vi "XML Script - GrowableNode (Style String).vi"(0 "x":i32=-1, 1 "y":i32=-1, 2 "out":i32=-1, 4 "Growable Node Style":string, 6 "name":string, 8 "size":i32=1, 9 "prefix (name)":string, 10 "in":i32=-1) -> (5 "name (wire source)":string, 7 "XML Script Command - Growable Node":string)   [LabVIEW 2017]
uses:
  <vilib>/_script/XML Scripting/XML Script Attribute.ctl
  <vilib>/_script/XML Scripting/XML Script Tag.ctl
panel:
  # "position"
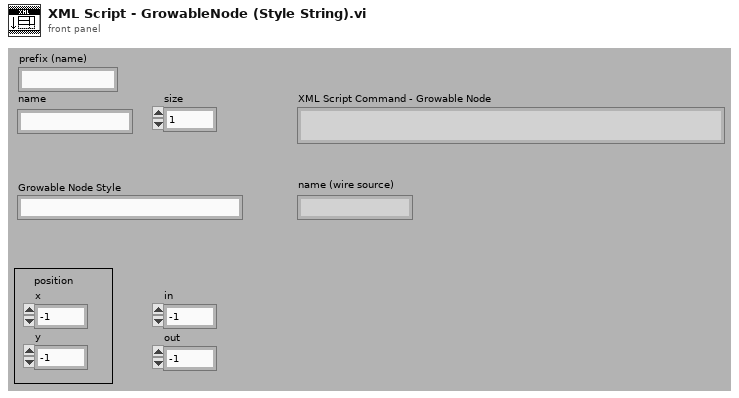
[diagram p1: front panel]
types:
  T1 = typedef "XML Script Attribute.ctl" = enum16{"name", "style", "path", "position", "in", "out", "width", "height", "index", "value", "default", "location", "offset", "typeindex", "size", "source", "destination", "indicator", "type", "controlname", "label", "conpaneidx", "mode", "description", "hasCondTerm", "linkIdentity", "caseselectortype", "concatInputs", "inName", "instantiationpath", "loopCondition", "IndexMode", "formulaInputs", "formulaOutputs", "msnFuncName", "msnIsDynamic", "msnIsODEUserFunction", "ignoreSearchDialog"}
  T2 = typedef "XML Script Tag.ctl" = enum16{"Script", "Function", "SubVI", "GrowableFunction", "Structure", "MultiframeStructure", "Frame", "Tunnel", "ShiftRegister", "Constant", "Control", "Terminal", "Wire", "StaticVIReference", "ControlTerminal", "CompoundArithmetic", "FlatSequence", "FlatSequenceFrame", "MathScriptCallByRef", "BuildArray", "GenericSubVI", "MathScriptNode"}
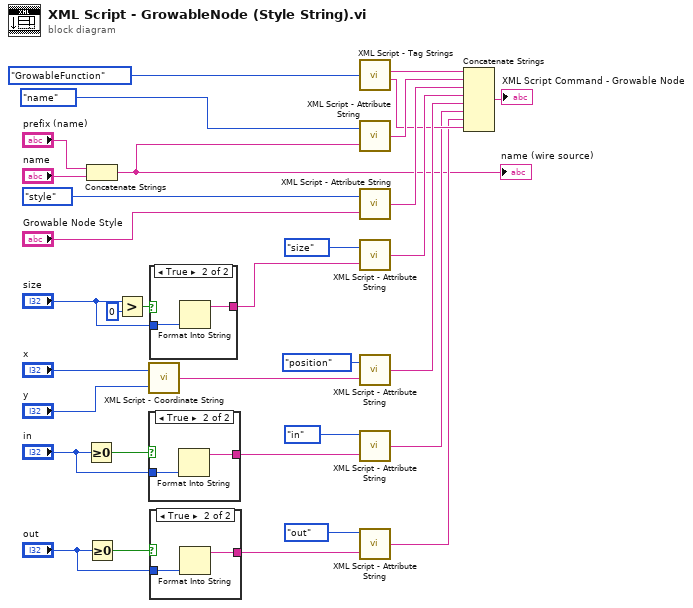
[diagram p0: block diagram]
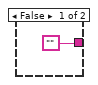
[diagram p2: hidden frame]
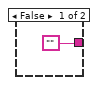
[diagram p3: hidden frame]
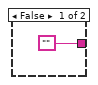
[diagram p4: hidden frame]
diagram:
  n1 = Greater Or Equal To 0?(x="in") -> (x >= 0?=w10:bool)
  n2 = Concatenate Strings("prefix (name)", "name") -> (w1:string)
  "name (wire source)" <- w1
  n3 = Greater Or Equal To 0?(x="out") -> (x >= 0?=w14:bool)
  n4 = Greater?(x="size", y=0) -> (0:w29:bool)
  n5 = call <vilib>:"XML Script - Coordinate String.vi"("y"="y", "x"="x") -> ("(x,y)"=w27:string)
  n6 = case shown="True" w10 {
    tunnel: "in" -> [_ w36]
    tunnel: ["" w35] -> w12
    frame False {
    }
    frame True {
      n7 = Format Into String(w36) -> (resulting string=w35:string)  [unwired: 3 in, 1 out]
    }
  }
  n8 = case shown="True" w29 {
    tunnel: "size" -> [_ w39]
    tunnel: ["" w38] -> w19
    frame False {
    }
    frame True {
      n9 = Format Into String(w39) -> (resulting string=w38:string)  [unwired: 3 in, 1 out]
    }
  }
  n10 = case shown="True" w14 {
    tunnel: "out" -> [_ w42]
    tunnel: ["" w41] -> w16
    frame False {
    }
    frame True {
      n11 = Format Into String(w42) -> (resulting string=w41:string)  [unwired: 3 in, 1 out]
    }
  }
  n12 = call <vilib>:"XML Script - Tag Strings.vi"("XML Script Tag"=XML_Script_Tag."GrowableFunction") -> ("XML String - Begin Tag"=w24:string, "XML String - End Tag"=w6:string)  [unwired: 2 in]
  n13 = call <vilib>:"XML Script - Attribute String.vi"("Attribute String"=w1, "XML Script Attribute"=XML_Script_Attribute."name") -> ("XML Script - Attribute String"=w22:string)
  n14 = call <vilib>:"XML Script - Attribute String.vi"("Attribute String"="Growable Node Style", "XML Script Attribute"=XML_Script_Attribute."style") -> ("XML Script - Attribute String"=w20:string)
  n15 = call <vilib>:"XML Script - Attribute String.vi"("Attribute String"=w19, "XML Script Attribute"=XML_Script_Attribute."size") -> ("XML Script - Attribute String"=w8:string)
  n16 = call <vilib>:"XML Script - Attribute String.vi"("Attribute String"=w27, "XML Script Attribute"=XML_Script_Attribute."position") -> ("XML Script - Attribute String"=w7:string)
  n17 = call <vilib>:"XML Script - Attribute String.vi"("Attribute String"=w12, "XML Script Attribute"=XML_Script_Attribute."in") -> ("XML Script - Attribute String"=w5:string)
  n18 = call <vilib>:"XML Script - Attribute String.vi"("Attribute String"=w16, "XML Script Attribute"=XML_Script_Attribute."out") -> ("XML Script - Attribute String"=w4:string)
  n19 = Concatenate Strings(w24, w22, w20, w8, w7, w5, w4, w6) -> (→"XML Script Command - Growable Node":string)
